vi "read field.vi"(8 "error in":errorcluster) -> (0 "error out":errorcluster, 2 "Current field (T)":dbl[unit])   [LabVIEW 2009, in "Varian Magnet.lvclass"]
uses:
  Varian Magnet.lvclass
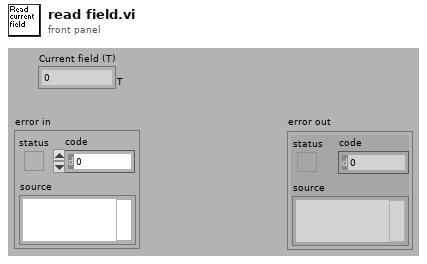
[diagram p1: front panel]
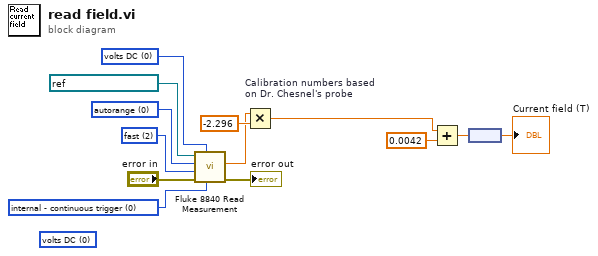
[diagram p0: block diagram]
diagram:
  w2 = u16 0 items=["volts DC", "volts AC", "2-wire k.ohms", "4-wire k.ohms", "mA DC", "mA AC"] ("function (0:volts DC)")
  w8 = u16 0 items=["internal - continuous trigger", "external - rear panel trigger with delay", "external - bus trigger with delay", "external - rear panel trigger", "external - bus trigger"] ("trigger mode (0:internal)")
  (unwired) u16 0 items=["volts DC", "volts AC", "2-wire k.ohms", "4-wire k.ohms", "mA DC", "mA AC"] ("function (0:volts DC)")
  w7 = u16 2 items=["slow", "medium", "fast"] ("rate (0:slow)")
  w6 = u16 0 items=["autorange", "200mV, 200 ohms", "2V, 2 kohms", "20V, 20 kohms", "200V, 200 kohms", "1000Vdc, 700 Vac, 2 Mohms", "20 Mohms"] ("range (0:auto)")
  n1 = call "Fluke 8840 Read Measurement.vi"("trigger mode (0:internal)"=w8, "function (0:volts DC)"=w2, "error in (no error)"="error in", "rate (0:slow)"=w7, "range (0:auto)"=w6, "VISA resource name"=refnum<visa-resource-name> "GPIB0::2::INSTR") -> ("error out"=→"error out":errorcluster, "measurement"=w1:dbl)  [unwired: 4 out]
  n2 = Multiply "Calibration numbers based\non Dr. Chesnel's probe"(x=w1, y=-2.296) -> (x*y=w12:dbl)
  n3 = Add(x=w12, y=0.0042 ("x")) -> (x+y=w11:dbl)
  n4 = node(w11) -> (→"Current field (T)":dbl[unit])
